vi "Parallax PING Read Distance.vi"(8 "error in (no error)":errorcluster, 10 "Temperature (deg C)":dbl=25.0, 11 "myRIO DIO Channel":tag="C/DIO1") -> (0 "error out":errorcluster, 3 "Distance (cm)":dbl)   [LabVIEW 2016]
doc: "Reads the distance in meters from the Parallax PING sensor located on the given pin.\n\nReturns -1 if the distance could not be read."
uses:
  <vilib>/myRIO/Instrument Drivers/Onboard IO/DIO/typedefs/DIO Reference.ctl
  <vilib>/myRIO/Common/Instrument Driver Framework/Utilities/typedefs/myRIO Generic Hardware Reference.ctl
  <vilib>/myRIO/Common/Instrument Driver Framework/Utilities/typedefs/Hardware Version Enum.ctl
  <vilib>/myRIO/Common/Instrument Driver Framework/Utilities/typedefs/myRIO v1.0 Reference.ctl
  <vilib>/myRIO/Common/Instrument Driver Framework/Utilities/typedefs/Generic FPGA Reference.ctl
  <vilib>/myRIO/Common/Instrument Driver Framework/myRIO v1.0/DIO/typedefs/DIO Channels List.ctl
  <vilib>/myRIO/Common/Instrument Driver Framework/myRIO v1.0/DIO/typedefs/DIO Channels Enum.ctl
  <vilib>/myRIO/Common/Instrument Driver Framework/myRIO v1.0/DIO/vis/myRIO v1.0 Close DIO.vi
  <vilib>/myRIO/Common/Instrument Driver Framework/myRIO v1.0/DIO/vis/myRIO v1.0 Unreserve DIO.vi
  <vilib>/myRIO/Common/Instrument Driver Framework/myRIO v1.0/DIO/vis/myRIO v1.0 Build MUX Configuration DIO.vi
  <vilib>/myRIO/Common/Instrument Driver Framework/myRIO v1.0/Resource Manager/vis/myRIO v1.0 Unreserve Channel List.vi
  <vilib>/myRIO/Common/Instrument Driver Framework/myRIO v1.0/Resource Manager/vis/myRIO v1.0 Create Configuration List.vi
  <vilib>/myRIO/Common/Instrument Driver Framework/myRIO v1.0/Resource Manager/vis/myRIO v1.0 Unreserve Channel.vi
  <vilib>/myRIO/Common/Instrument Driver Framework/myRIO v1.0/Resource Manager/vis/myRIO v1.0 Build Mutex Name.vi
  <vilib>/Utility/error.llb/Error Cluster From Error Code.vi
  <vilib>/myRIO/Common/Instrument Driver Framework/myRIO v1.0/myRIO v1.0 Close.vi
  <vilib>/myRIO/Common/Instrument Driver Framework/Utilities/vis/IO Manager.vi
  <vilib>/myRIO/Common/Instrument Driver Framework/Utilities/vis/Configuration Manager.vi
  <vilib>/myRIO/Common/Instrument Driver Framework/myRIO v1.0/Resource Manager/vis/myRIO v1.0 Configure IO.vi
  <vilib>/myRIO/Common/Instrument Driver Framework/myRIO v1.0/DIO/vis/myRIO v1.0 Shutdown DIO.vi
  <vilib>/myRIO/Common/Instrument Driver Framework/myRIO v1.0/DIO/vis/myRIO v1.0 Read DIO.vi
  <vilib>/myRIO/Common/Instrument Driver Framework/myRIO v1.0/DIO/vis/myRIO v1.0 Write DIO.vi
  <vilib>/myRIO/Instrument Drivers/Onboard IO/DIO/DIO.lvlib
panel:
  in  "stop":bool
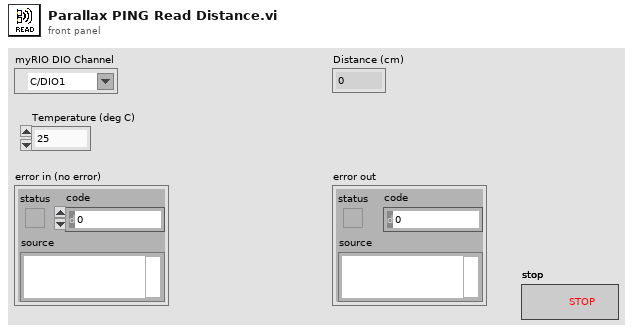
[diagram p1: front panel]
types:
  T1 = enum16{"Initialize", "Trigger pulse", "Wait for rising edge", "Wait for falling edge", "Calculate distance", "Stop"}
  T2 = typedef "DIO.lvlib/DIO Reference.ctl" = cluster{"myRIO Reference":T3, "DIO Channels List":T7}
  T3 = typedef "myRIO Generic Hardware Reference.ctl" = cluster{"myRIO Model":T4, "myRIO Hardware Reference":T5}
  T4 = typedef "Hardware Version Enum.ctl" = enum16{"Unknown", "myRIO-1900", "myRIO-1950", "roboRIO", "NI ELVIS RIO CM"}
  T5 = typedef "myRIO v1.0 Reference.ctl" = cluster{"Generic FPGA Reference":T6, "Allow multiple opens":bool}
  T6 = typedef "Generic FPGA Reference.ctl" = refnum<k20>
  T7 = typedef "DIO Channels List.ctl" = T8[]
  T8 = typedef "DIO Channels Enum.ctl" = enum16{"Not Connected", "C/DIO0", "C/DIO1", "C/DIO2", "C/DIO3", "C/DIO4", "C/DIO5", "C/DIO6", "C/DIO7", "A/DIO0", "A/DIO1", "A/DIO2", "A/DIO3", "A/DIO4", "A/DIO5", "A/DIO6", "A/DIO7", "A/DIO8", "A/DIO9", "A/DIO10", "A/DIO11", "A/DIO12", "A/DIO13", "A/DIO14", "A/DIO15", "B/DIO0", "B/DIO1", "B/DIO2", "B/DIO3", "B/DIO4", "B/DIO5", "B/DIO6", "B/DIO7", "B/DIO8", "B/DIO9", "B/DIO10", "B/DIO11", "B/DIO12", "B/DIO13", "B/DIO14", "B/DIO15", "LED0", "LED1", "LED2", "LED3", "Button0", "DIO/DIO0", "DIO/DIO1", "DIO/DIO2", "DIO/DIO3", "DIO/DIO4", "DIO/DIO5", "DIO/DIO6", "DIO/DIO7", "DIO/DIO8", "DIO/DIO9", "SPI/CS0", "SPI/CS1", "SPI/CS2", "SPI/CS3", "LED RADIO (Green)", "LED RADIO (Red)", "LED COMM (Green)", "LED COMM (Red)", "LED MODE (Green)", "LED MODE (Red)"}
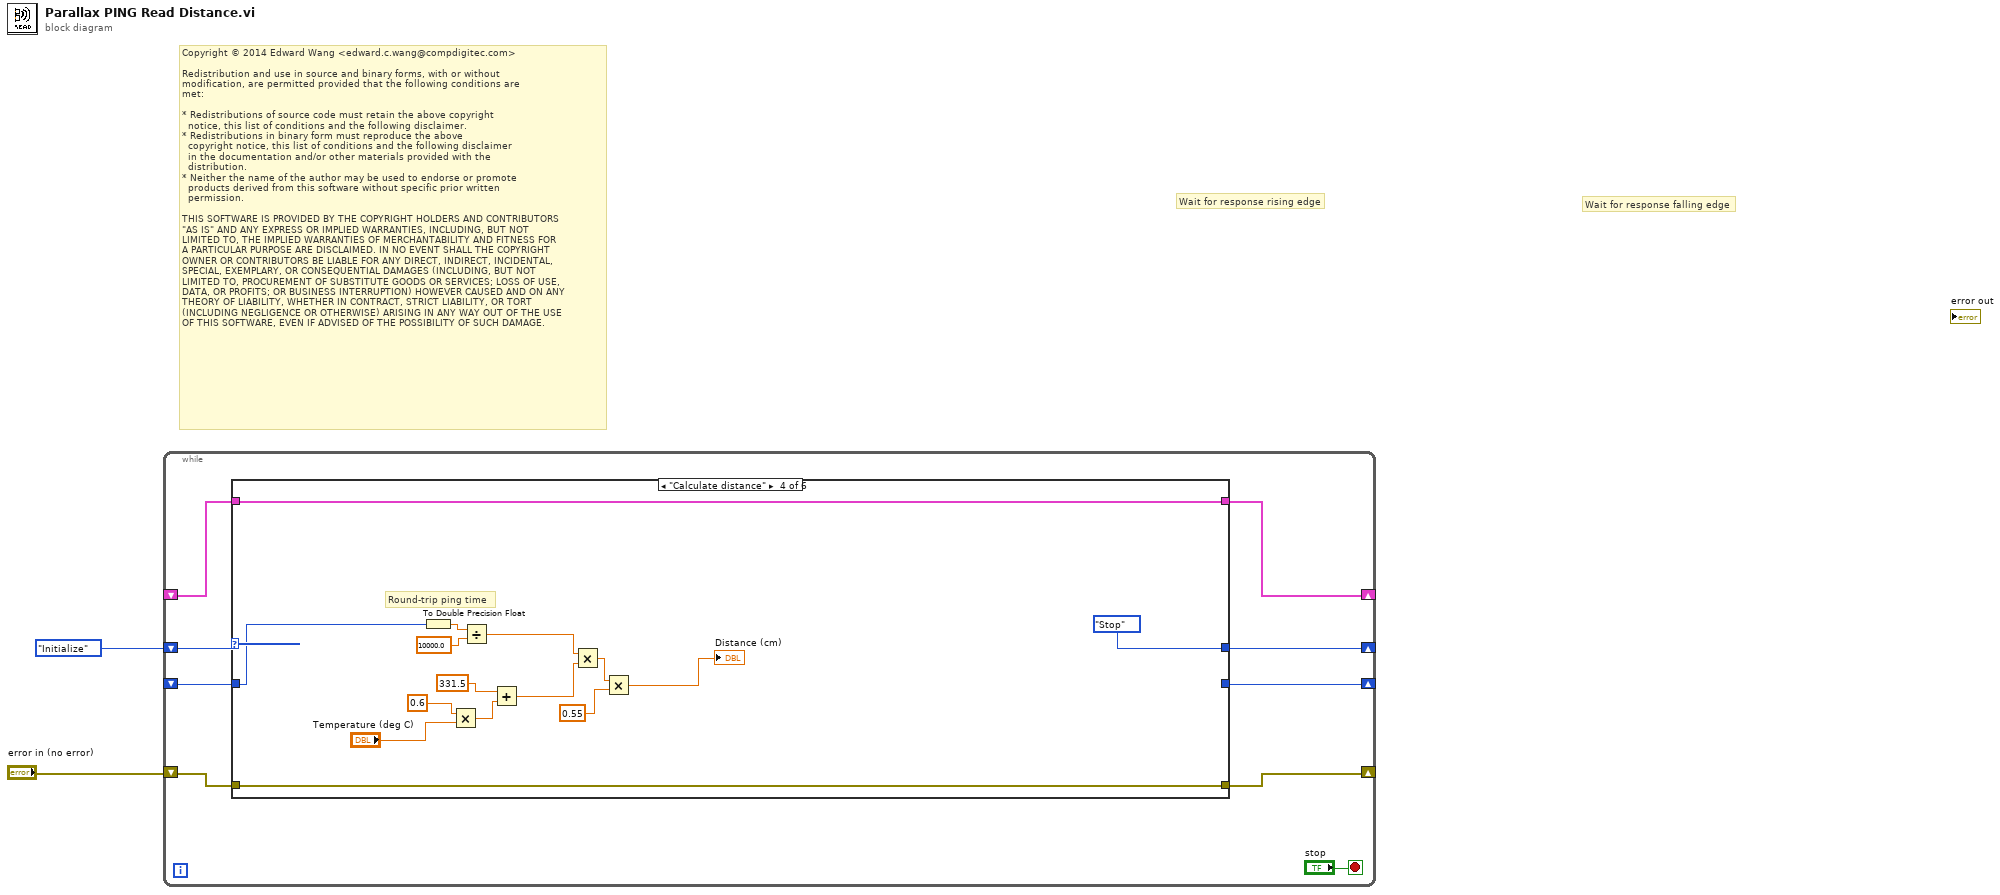
[diagram p0: block diagram]
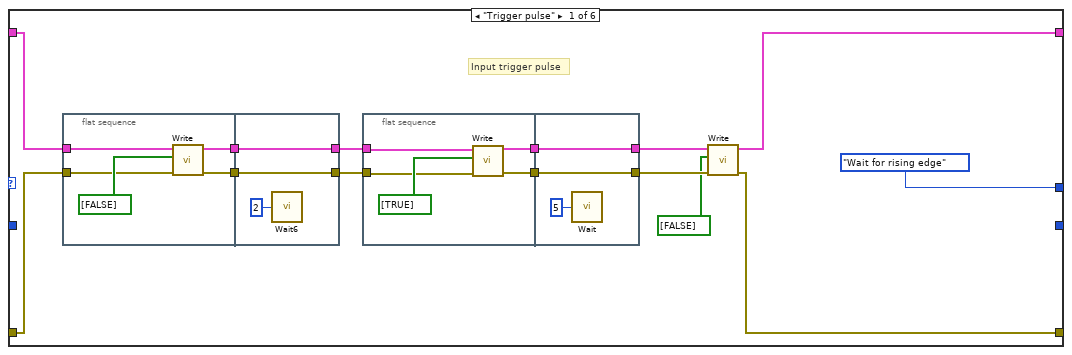
[diagram p2: hidden frame]
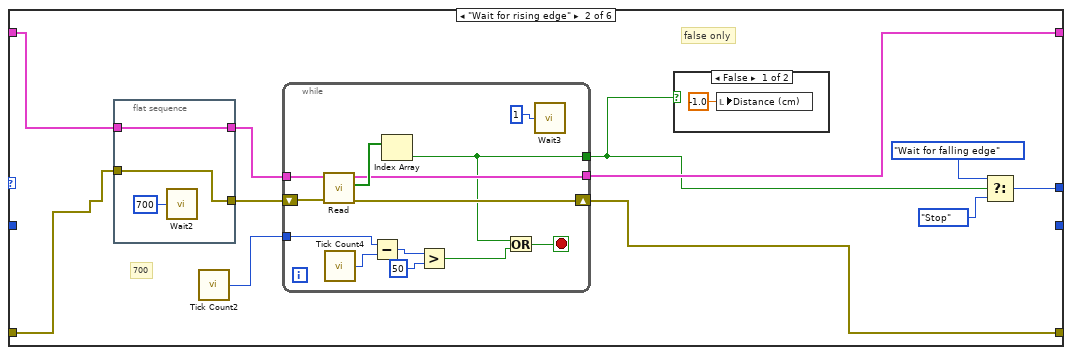
[diagram p3: hidden frame]
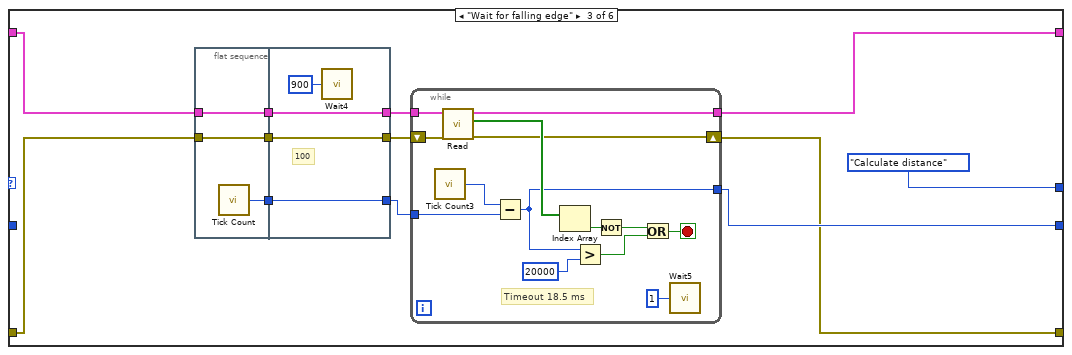
[diagram p5: hidden frame]
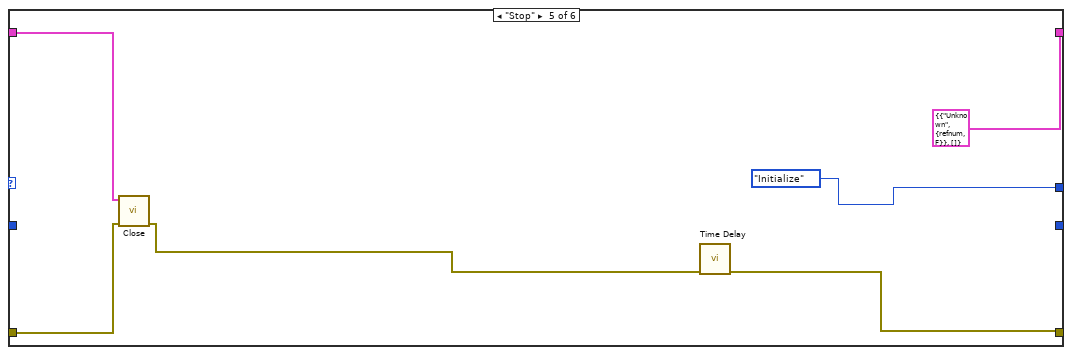
[diagram p6: hidden frame]
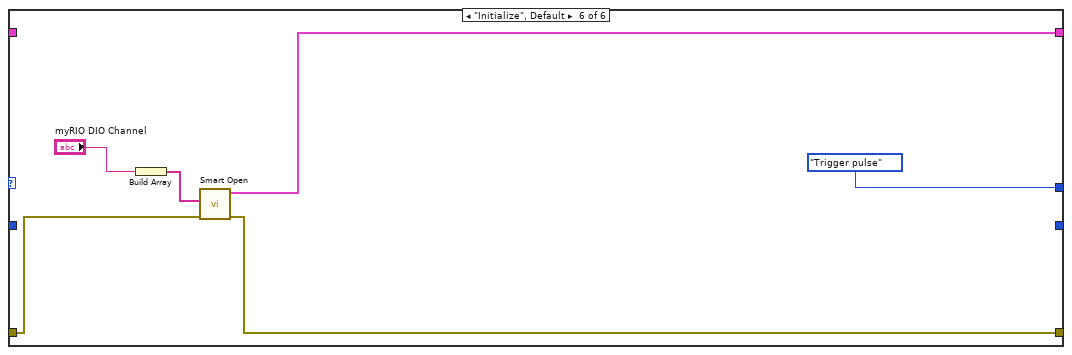
[diagram p7: hidden frame]
diagram:
  # "Copyright © 2014 Edward Wang <edward.c.wang@compdigitec.com>\n\nRedistribution and use in source and binary forms, with or without\nmodification, are permitted provided that the following conditions are\nmet:\n\n* Redistributions of source code must retain the above copyright\n  notice, this list of conditions and the following disclaimer.\n* Redistributions in binary form must reproduce the above\n  copyright notice, this list of conditions and the following disclaimer\n  in the documentation and/or other materials provided with the\n  distribution.\n* Neither the name of the author may be used to endorse or promote\n  products derived from this software without specific prior written\n  permission.\n\nTHIS SOFTWARE IS PROVIDED BY THE COPYRIGHT HOLDERS AND CONTRIBUTORS\n\"AS IS\" AND ANY EXPRESS OR IMPLIED WARRANTIES, INCLUDING, BUT NOT\nLIMITED TO, THE IMPLIED WARRANTIES OF MERCHANTABILITY AND FITNESS FOR\nA PARTICULAR PURPOSE ARE DISCLAIMED. IN NO EVENT SHALL THE COPYRIGHT\nOWNER OR CONTRIBUTORS BE LIABLE FOR ANY DIRECT, INDIRECT, INCIDENTAL,\nSPECIAL, EXEMPLARY, OR CONSEQUENTIAL DAMAGES (INCLUDING, BUT NOT\nLIMITED TO, PROCUREMENT OF SUBSTITUTE GOODS OR SERVICES; LOSS OF USE,\nDATA, OR PROFITS; OR BUSINESS INTERRUPTION) HOWEVER CAUSED AND ON ANY\nTHEORY OF LIABILITY, WHETHER IN CONTRACT, STRICT LIABILITY, OR TORT\n(INCLUDING NEGLIGENCE OR OTHERWISE) ARISING IN ANY WAY OUT OF THE USE\nOF THIS SOFTWARE, EVEN IF ADVISED OF THE POSSIBILITY OF SUCH DAMAGE."
  # "Wait for response falling edge"
  # "Wait for response rising edge"
  n1 = while {
    shift-right: [w5] -> _
    shift-left: T1."Initialize" -> [w11]
    shift-right: [w7] -> _
    shift-left: "error in (no error)" -> [w10]
    shift-right: [w9] -> _
    shift-left: _ -> [w8]
    shift-right: [w3] -> _
    shift-left: _ -> [w6]
    stop <- "stop" stop-if-true
    n2 = case shown="\"Calculate distance\"" w11 {
      tunnel: [T1."Wait for rising edge" w43 T1."Calculate distance" ("y") T1."Stop" ("y") T1."Initialize" ("y") T1."Trigger pulse"] -> w5
      tunnel: w10 -> [w16 w48 w74 w105 w123 w127]
      tunnel: [w14 w52 w73 w117 T2 {"myRIO Reference"={"myRIO Model"=enum."Unknown", "myRIO Hardware Reference"={"Generic FPGA Reference"=refnum, "Allow multiple opens"=FALSE}}, "DIO Channels List"=[]} ("DIO Ref Out") w126] -> w9
      tunnel: w8 -> [w15 w47 w75 w117 w122 _]
      tunnel: [w13 w51 w70 w105 w118 w125] -> w7
      tunnel: [_ _ w72 _ _ _] -> w3
      tunnel: w6 -> [_ _ _ w104 _ _]
      frame "Trigger pulse" {
        # "Input trigger pulse"
        n3 = flat-sequence {
          tunnel: [w29] -> w23
          tunnel: [w28] -> w22
          tunnel: w16 -> [w27]
          tunnel: w15 -> [w26]
          tunnel: [w32] -> w20
          tunnel: [w31] -> w21
          tunnel: w23 -> [w32]
          tunnel: w22 -> [w31]
          frame #0 {
            n4 = call <vilib>:"Write.vi"("error in (no error)"=w27, "Values"=bool[] [FALSE], "DIO Ref In"=w26) -> ("error out"=w28:errorcluster, "DIO Ref Out"=w29:T2)  [unwired: 6 in]
          }
          frame #1 {
            n5 = call "Wait6"("Count(uSec)"=u32 2) -> ()  [unwired: 1 out]
          }
        }
        n6 = flat-sequence {
          tunnel: [w37] -> w25
          tunnel: [w36] -> w24
          tunnel: w21 -> [w35]
          tunnel: w20 -> [w34]
          tunnel: [w40] -> w17
          tunnel: [w39] -> w19
          tunnel: w25 -> [w40]
          tunnel: w24 -> [w39]
          frame #0 {
            n7 = call <vilib>:"Write.vi"("error in (no error)"=w35, "Values"=bool[] [TRUE], "DIO Ref In"=w34) -> ("error out"=w36:errorcluster, "DIO Ref Out"=w37:T2)  [unwired: 6 in]
          }
          frame #1 {
            n8 = call "Wait"("Count(uSec)"=u32 5) -> ()  [unwired: 1 out]
          }
        }
        n9 = call <vilib>:"Write.vi"("error in (no error)"=w19, "Values"=bool[] [FALSE], "DIO Ref In"=w17) -> ("error out"=w13:errorcluster, "DIO Ref Out"=w14:T2)  [unwired: 6 in]
      }
      frame "Wait for rising edge" {
        # "700"
        # "false only"
        n10 = flat-sequence {
          tunnel: [w55] -> w49
          tunnel: w48 -> [w55]
          tunnel: w47 -> [w54]
          tunnel: [w54] -> w46
          frame #0 {
            n11 = call "Wait2"("Count(uSec)"=u32 700) -> ()  [unwired: 1 out]
          }
        }
        n12 = call "Tick Count2"() -> ("Tick Count(uSec)"=w50:u32)
        n13 = while {
          tunnel: [w67] -> w52
          shift-right: [w65] -> w51
          shift-left: w49 -> [w66]
          tunnel: w50 -> [w62]
          tunnel: w46 -> [w64]
          tunnel: [w57] -> w42
          stop <- w59 stop-if-true
          n14 = call <vilib>:"Read.vi"("error in (no error)"=w66, "DIO Ref In"=w64) -> ("error out"=w65:errorcluster, "Values"=w68:bool[], "DIO Ref Out"=w67:T2)  [unwired: 7 in]
          n15 = call "Tick Count4"() -> ("Tick Count(uSec)"=w63:u32)
          n16 = Subtract(x=w62, y=w63) -> (x-y=w61:u32)
          n17 = Index Array(array=w68) -> (element=w57:bool)  [unwired: 1 in]
          n18 = Greater?(x=w61, y=u32 50) -> (0:w58:bool)
          n19 = Or(x=w57, y=w58) -> (x .or. y?=w59:bool)
          n20 = call "Wait3"("Count(uSec)"=u32 1) -> ()  [unwired: 1 out]
        }
        n21 = case shown="False" w42 {
          frame False {
            n22 = local write "Distance (cm)"(-1.0 ("Distance (m)")) -> ()
          }
          frame True {
          }
        }
        n23 = Select(t=T1."Wait for falling edge", s=w42, f=T1."Stop" ("y")) -> (s? t:f=w43:T1)
      }
      frame "Wait for falling edge" {
        n24 = flat-sequence {
          tunnel: w75 -> [w98]
          tunnel: [w98] -> w81
          tunnel: [w97] -> w80
          tunnel: [w96] -> w79
          tunnel: w74 -> [w96]
          tunnel: [w101] -> w77
          tunnel: [w102] -> w78
          tunnel: w81 -> [w102]
          tunnel: w80 -> [w101]
          tunnel: w79 -> [w99]
          tunnel: [w99] -> w76
          frame #0 {
            n25 = call "Tick Count"() -> ("Tick Count(uSec)"=w97:u32)
          }
          frame #1 {
            # "100"
            n26 = call "Wait4"("Count(uSec)"=u32 900) -> ()  [unwired: 1 out]
          }
        }
        n27 = while {
          tunnel: w78 -> [w94]
          tunnel: w77 -> [w91]
          shift-right: [w85] -> w70
          shift-left: w76 -> [w86]
          tunnel: [w83] -> w73
          tunnel: [w82] -> w72
          stop <- w90 stop-if-true
          # "Timeout 18.5 ms"
          n28 = call "Tick Count3"() -> ("Tick Count(uSec)"=w84:u32)
          n29 = call <vilib>:"Read.vi"("error in (no error)"=w86, "DIO Ref In"=w94) -> ("error out"=w85:errorcluster, "Values"=w93:bool[], "DIO Ref Out"=w83:T2)  [unwired: 7 in]
          n30 = Subtract(x=w84, y=w91) -> (x-y=w82:u32)
          n31 = Index Array(array=w93) -> (element=w92:bool)  [unwired: 1 in]
          n32 = Greater?(x=w82, y=u32 20000) -> (0:w88:bool)
          n33 = Not(x=w92) -> (.not. x?=w89:bool)
          n34 = Or(x=w89, y=w88) -> (x .or. y?=w90:bool)
          n35 = call "Wait5"("Count(uSec)"=u32 1) -> ()  [unwired: 1 out]
        }
      }
      frame "Calculate distance" {
        # "Round-trip ping time"
        n36 = To Double Precision Float(number=w104) -> (double precision float=w112:dbl)
        n37 = Multiply(x=0.6, y="Temperature (deg C)") -> (x*y=w110:dbl)
        n38 = Divide(x=w112, y=10000.0) -> (x/y=w114:dbl)
        n39 = Add(x=331.5, y=w110) -> (x+y=w115:dbl)
        n40 = Multiply(x=w114, y=w115) -> (x*y=w107:dbl)
        n41 = Multiply(x=w107, y=0.55) -> (x*y=→"Distance (cm)":dbl)
      }
      frame "Stop" {
        n42 = call <vilib>:"Close.vi"("error in (no error)"=w123, "DIO Ref In"=w122) -> ("error out"=w119:errorcluster)  [unwired: 9 in]
        n43 = call "Time Delay"("error in (no error)"=w119) -> ("error out"=w118:errorcluster)  [unwired: 10 in]
      }
      frame "Initialize", Default {
        n44 = Build Array("myRIO DIO Channel") -> (w129:tag[])
        n45 = call <vilib>:"Smart Open.vi"("error in (no error)"=w127, "Channel Names"=w129) -> ("error out"=w125:errorcluster, "DIO Ref Out"=w126:T2)  [unwired: 8 in]
      }
    }
  }
